vi "Delete CSM Module.vi"(6 "Config Path":path, 8 "error in (no error)":errorcluster, 11 "CSM Name":string) -> (0 "error out":errorcluster)   [LabVIEW 2017, in "CSM-Helper API with lvcsm Support.lvlib"]
uses:
  CSM-Helper API with lvcsm Support.lvlib
  <vilib>/Utility/config.llb/NI_LVConfig.lvlib
  lvcsmFile/lvcsm File Support.lvlib
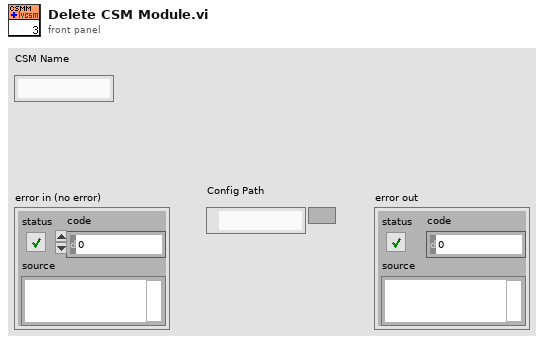
[diagram p1: front panel]
types:
  T1 = typedef "NI_LVConfig.lvlib/Config Data RefNum.ctl" = refnum<k1>
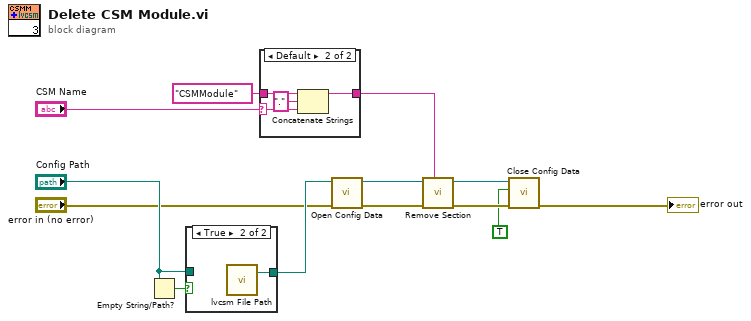
[diagram p0: block diagram]
diagram:
  n1 = Empty String/Path?(string/path="Config Path") -> (empty?=w11:bool)
  n2 = case shown="True" w11 {
    tunnel: [w14 w15] -> w13
    tunnel: "Config Path" -> [w14 _]
    frame False {
    }
    frame True {
      n3 = call "lvcsm File Path.vi"() -> ("Appended Path"=w15:path)  [unwired: 3 in]
    }
  }
  n4 = case shown="Default" "CSM Name" {
    selector: "CSM Name" -> [_ w18]
    tunnel: "CSMModule" ("Section Prefix") -> [w16 w20]
    tunnel: [w16 w19] -> w6
    frame "" {
    }
    frame Default {
      n5 = Concatenate Strings(w20, "." ("string"), w18) -> (w19:string)
    }
  }
  n6 = call <vilib>:"Open Config Data.vi"("error in (no error)"="error in (no error)", "configuration file path"=w13) -> ("error out"=w2:errorcluster, "refnum"=w3:T1)  [unwired: 7 in, 1 out]
  n7 = call <vilib>:"Remove Section.vi"("section"=w6, "error in (no error)"=w2, "refnum"=w3) -> ("error out"=w4:errorcluster, "refnum out"=w5:T1)  [unwired: 6 in, 1 out]
  n8 = call <vilib>:"Close Config Data.vi"("error in (no error)"=w4, "write file if changed (T)"=TRUE, "refnum"=w5) -> ("error out"=→"error out":errorcluster)  [unwired: 7 in, 1 out]
